vi "CANdleSetter.vi"   [LabVIEW 2025]
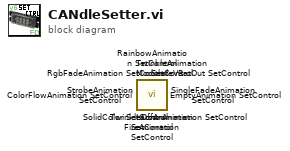
[diagram p0: block diagram]
diagram:
  n1 = call <vilib>:"TwinkleOffAnimation SetControl.vi"() -> ()  [unwired: 26 in, 2 out]
  n2 = call <vilib>:"TwinkleAnimation SetControl.vi"() -> ()  [unwired: 26 in, 2 out]
  n3 = call <vilib>:"StrobeAnimation SetControl.vi"() -> ()  [unwired: 26 in, 2 out]
  n4 = call <vilib>:"SingleFadeAnimation SetControl.vi"() -> ()  [unwired: 26 in, 2 out]
  n5 = call <vilib>:"RgbFadeAnimation SetControl.vi"() -> ()  [unwired: 26 in, 2 out]
  n6 = call <vilib>:"RainbowAnimation SetControl.vi"() -> ()  [unwired: 26 in, 2 out]
  n7 = call <vilib>:"LarsonAnimation SetControl.vi"() -> ()  [unwired: 26 in, 2 out]
  n8 = call <vilib>:"FireAnimation SetControl.vi"() -> ()  [unwired: 26 in, 2 out]
  n9 = call <vilib>:"ColorFlowAnimation SetControl.vi"() -> ()  [unwired: 26 in, 2 out]
  n10 = call <vilib>:"EmptyAnimation SetControl.vi"() -> ()  [unwired: 26 in, 2 out]
  n11 = call <vilib>:"SolidColor SetControl.vi"() -> ()  [unwired: 26 in, 2 out]
  n12 = call <vilib>:"ModulateVBatOut SetControl.vi"() -> ()  [unwired: 26 in, 2 out]
